vi "Write.vi"(6 "Mask payload?":bool, 7 "timeout ms (5000)":i32=5000, 8 "error in (no error)":errorcluster, 9 "Data Format (Text)":T1, 10 "Data":string, 11 "WebSocket Connection in":refnum<k5>) -> (0 "error out":errorcluster, 3 "WebSocket Connection out":refnum<k5>)   [LabVIEW 2017, in "LV WebSockets.lvlib"]
doc: "Sends a WebSocket message to the client, either in text or binary format. Messages sent from the client must be masked but it is optional for the server.\nWebSockets 1.6.0.22\nSam Sharp - MediaMongrels Ltd\nCopyright (c) 2016, MediaMongrels Ltd"
uses:
  LV WebSockets.lvlib
  Data Format.ctl
  Opcode.ctl
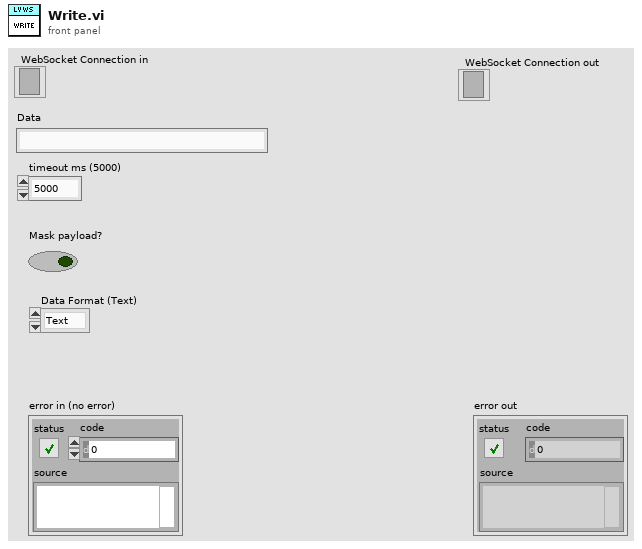
[diagram p1: front panel]
types:
  T1 = typedef "LV WebSockets.lvlib/Data Format.ctl" = enum16{"Text", "Binary"}
  T2 = typedef "LV WebSockets.lvlib/Opcode.ctl" = enum8{"Continuation Frame", "Text Frame", "Binary Frame", "Reserved 3", "Reserved 4", "Reserved 5", "Reserved 6", "Reserved 7", "Connection Close", "Ping", "Pong", "Reserved B", "Reserved C", "Reserved D", "Reserved F"}
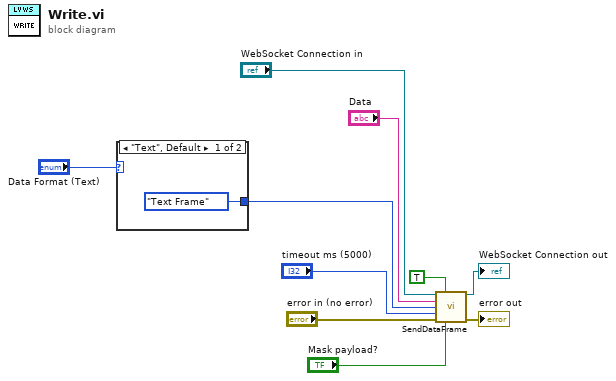
[diagram p0: block diagram]
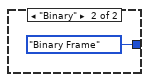
[diagram p2: hidden frame]
diagram:
  n1 = case shown="\"Text\", Default" "Data Format (Text)" {
    tunnel: [Opcode."Text Frame" ("Opcode") Opcode."Binary Frame" ("Opcode")] -> w8
    frame "Text", Default {
    }
    frame "Binary" {
    }
  }
  n2 = call "SendDataFrame.vi"("WebSocket Connection in"="WebSocket Connection in", "Final Frame Bit  (F)"=TRUE ("FIN Bit (F)"), "Data"="Data", "Opcode"=w8, "timeout ms (5000)"="timeout ms (5000)", "error in (no error)"="error in (no error)", "Mask payload?"="Mask payload?") -> ("WebSocket Connection out"=→"WebSocket Connection out":refnum<k5>, "error out"=→"error out":errorcluster)  [unwired: 7 in]
